vi "MoveJoints.vi"(0 "error in (no error)":errorcluster, 5 "HighSpeedEServer":refnum<k24>, 7 "axesPulse":i32[](array[numeric]), 9 "Speed":cluster{"classification":i32, "speed":dbl} {"classification" items=["LinkPercent", "Cartesian_MM_S", "Cartesian_DEG_S"]}, 11 "commandtype":i32(ring)=1 items=["LinkAbsolute"=1, "StraightAbsolute"=2, "StraightIncrement"=3]) -> (4 "error out":errorcluster)   [LabVIEW 2011, in "UnderAutomation.Yaskawa.lvlib"]
uses:
  UnderAutomation.Yaskawa.lvlib
  C:/Users/fg/Documents/Yaskawa.vi/LabVIEW_2024/UnderAutomation.Yaskawa/lib/UnderAutomation.Yaskawa.dll
  LabVIEW_2024/UnderAutomation.Yaskawa/lib/UnderAutomation.Yaskawa.dll
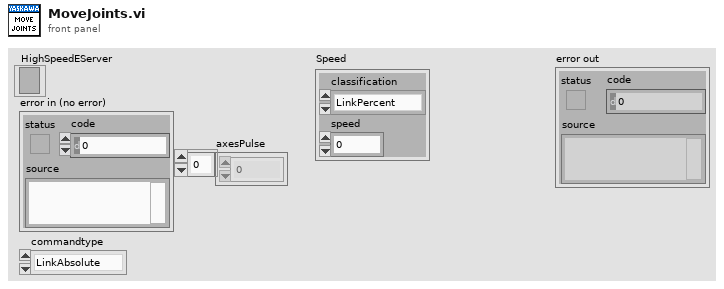
[diagram p1: front panel]
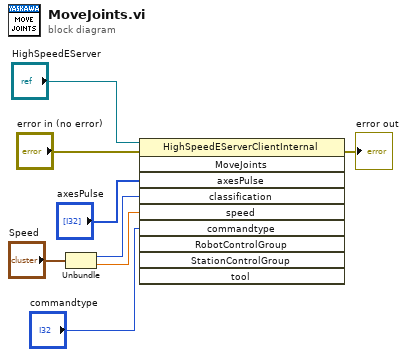
[diagram p0: block diagram]
diagram:
  n1 = Unbundle("Speed") -> ("classification"=w6:i32, "speed"=w2:dbl)
  n2 = invoke class="HighSpeedEServerClientInternal" method="MoveJoints"(reference="HighSpeedEServer", error in="error in (no error)", "axesPulse"="axesPulse", "classification"=w6, "speed"=w2, "commandtype"="commandtype") -> (error out=→"error out":errorcluster)  [unwired: 4 in, 9 out]
